vi "subVI.vi"() -> ()   [LabVIEW 2023]
panel:
  out "Posortowana macierz":dbl[][](array[numeric])
  in  "Y":dbl
  in  "X":dbl
  out "Macierz":dbl[][](array[numeric])
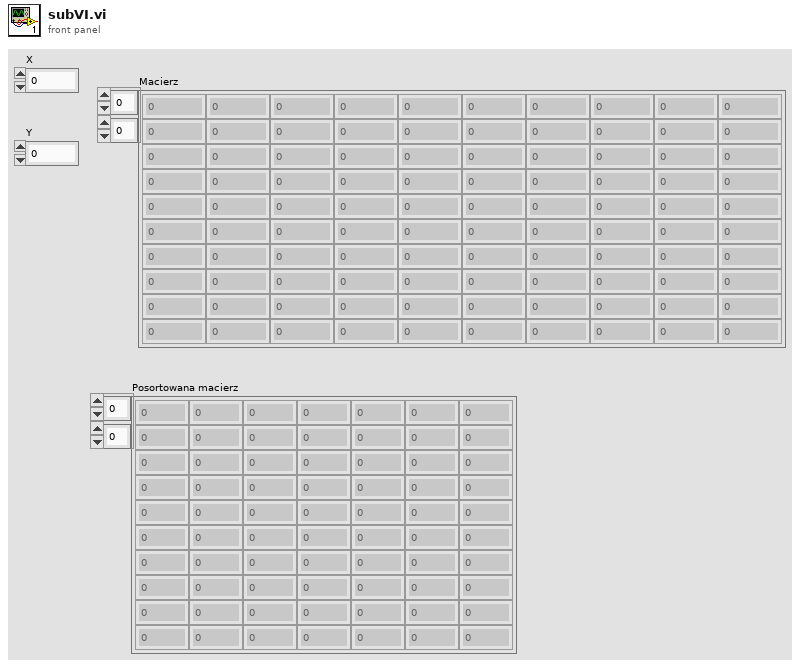
[diagram p1: front panel]
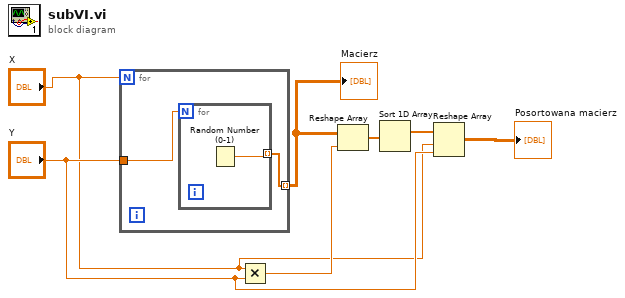
[diagram p0: block diagram]
diagram:
  n1 = for {
    N: "X" -> [_]
    tunnel: [w9] -> w7 mode=indexing
    tunnel: "Y" -> [w8]
    n2 = for {
      N: w8 -> [_]
      tunnel: [w10] -> w9 mode=indexing
      n3 = Random Number (0-1)() -> (number: 0 to 1=w10:dbl)
    }
  }
  "Macierz" <- w7
  n4 = Multiply(x="X", y="Y") -> (x*y=w4:dbl)
  n5 = Reshape Array(w7, w4) -> (w6:dbl[])
  n6 = Sort 1D Array(array=w6) -> (sorted array=w5:dbl[])
  n7 = Reshape Array(w5, "X", "Y") -> (→"Posortowana macierz":dbl[][])
